vi "Filter Compare.vi"(10 "quantized filter":T1 {"mSRate_QSettings"."source" items=["Coef a/k"=0, "Coef b/v"=7, "Input"=1, "Output"=2, "Multiplicand"=3, "Product"=4, "Sum"=5, "Delay"=6, "Gain"=8]}, 11 "filter":T1 {"mSRate_QSettings"."source" items=["Coef a/k"=0, "Coef b/v"=7, "Input"=1, "Output"=2, "Multiplicand"=3, "Product"=4, "Sum"=5, "Delay"=6, "Gain"=8]}) -> (2 "phase (deg)":cluster{"Y":dbl[], "Y":dbl[]}[](graph), 3 "gain (dB)":cluster{"Y":dbl[], "Y":dbl[]}[](graph))   [LabVIEW 2011]
uses:
  <vilib>/addons/Digital Filter Design/_Objects.llb/DFD Filter Obj.ctl
  <vilib>/addons/Digital Filter Design/_Objects.llb/DFD Filter Coef.ctl
  <vilib>/addons/Digital Filter Design/_Objects.llb/DFD Filter Structure Type Selector.ctl
  <vilib>/addons/Digital Filter Design/_Objects.llb/dfd_Internal Quantization Settings.ctl
  <vilib>/addons/Digital Filter Design/_Objects.llb/dfd_Internal Quantization Srcs.ctl
  <vilib>/addons/Digital Filter Design/_Objects.llb/DFD Coef Norm Type.ctl
  <vilib>/addons/Digital Filter Design/_Objects.llb/DFD Phase Setting.ctl
  <vilib>/addons/Digital Filter Design/NI_DigFilterLicensed.lvlib
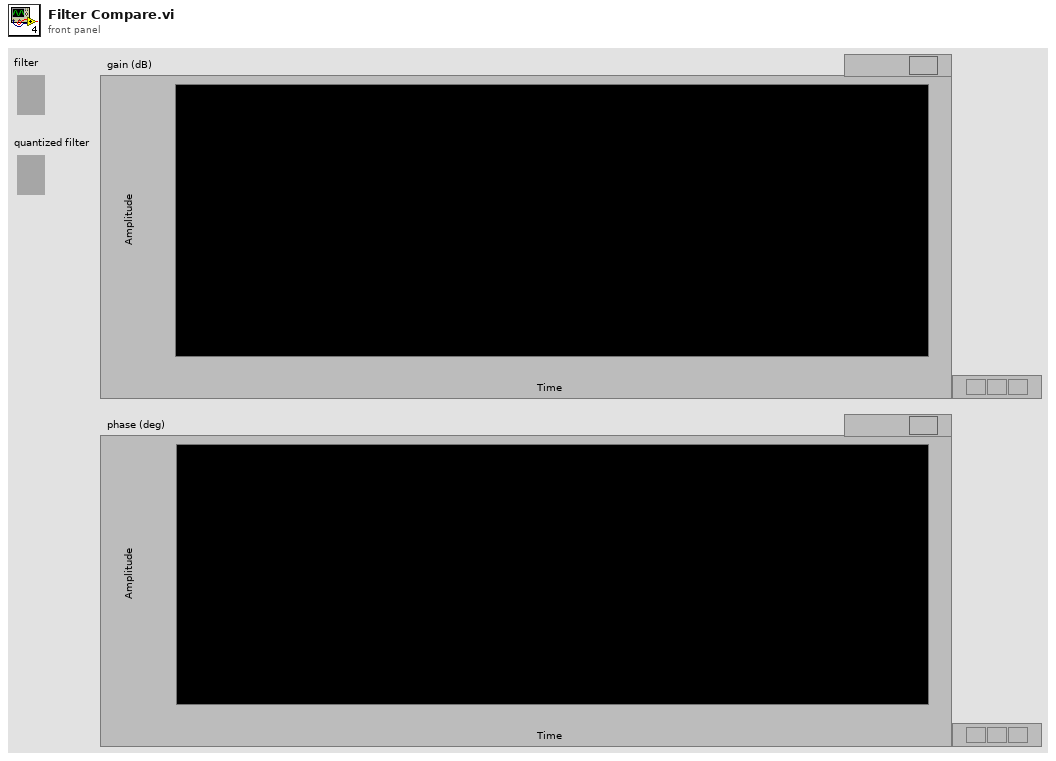
[diagram p1: front panel]
types:
  T1 = typedef "NI_DigFilterLicensed.lvlib/DFD Filter Obj.ctl" = cluster{"mSRate_Fs":dbl, "mSRate_Version":string, "mSRate_Comments":string, "mSRate_OrgCoef":T2, "mSRate_CurCoef":T2, "mSRate_Quantized?":bool, "mSRate_QCoef":T2, "mSRate_QSettings":T4[], "mSRate_Order":i32, "mSRate_Scaling":cluster{"mSRate_ScaleByPowerOf2?":bool, "mSRate_ScaleType":T6}}
  T2 = typedef "NI_DigFilterLicensed.lvlib/DFD Filter Coef.ctl" = cluster{"type":T3, "gain":dbl, "coef a (k)":dbl[], "coef b (v)":dbl[]}
  T3 = typedef "NI_DigFilterLicensed.lvlib/DFD Filter Structure Type Selector.ctl" = enum16{"Undefined", "FIR Direct Form", "FIR Direct Form Transposed", "FIR Symmetric", "FIR Antisymmetric", "IIR Direct Form I", "IIR Direct Form I Transposed", "IIR Direct Form II", "IIR Direct Form II Transposed", "IIR Cascaded Second Order Sections Form I", "IIR Cascaded Second Order Sections Form I Transposed", "IIR Cascaded Second Order Sections Form II", "IIR Cascaded Second Order Sections Form II Transposed", "Lattice Allpass (basic sections)", "Lattice Allpass (one multiplier sections)", "Lattice Allpass (normalized sections)", "Lattice AR (basic sections)", "Lattice AR (one multiplier sections)", "Lattice AR (normalized sections)", "Lattice MA (minimum phase)", "Lattice MA (maximum phase)", "Lattice ARMA (basic sections)", "Lattice ARMA (one multiplier sections)", "Lattice ARMA (normalized sections)"}
  T4 = typedef "NI_DigFilterLicensed.lvlib/dfd_Internal Quantization Settings.ctl" = cluster{"source":T5, "wl":i16, "iwl":i16, "overflow mode":enum16{"Saturation", "Wrap"}, "rounding mode":enum16{"Nearest", "Truncation"}, "signed?":bool}
  T5 = typedef "NI_DigFilterLicensed.lvlib/dfd_Internal Quantization Srcs.ctl" = u16
  T6 = typedef "NI_DigFilterLicensed.lvlib/DFD Coef Norm Type.ctl" = enum16{"No Norm", "Time Domain 1-Norm", "Time Domain 2-Norm", "Time Domain Inf-Norm"}
  T7 = typedef "NI_DigFilterLicensed.lvlib/DFD Phase Setting.ctl" = cluster{"unwrap? (F)":bool, "degree? (F)":bool}
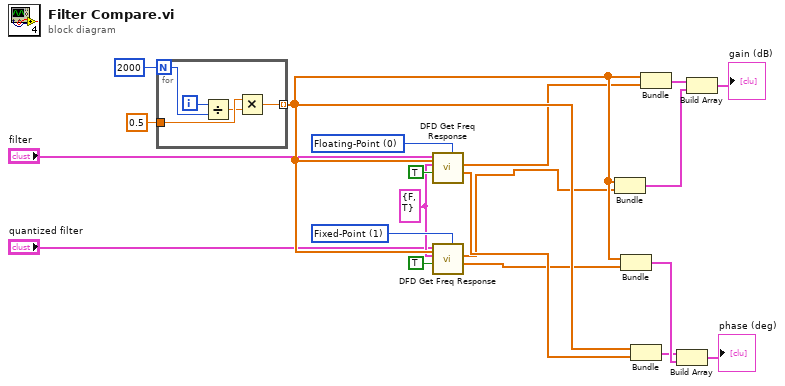
[diagram p0: block diagram]
diagram:
  w3 = T7 {"unwrap? (F)"=FALSE, "degree? (F)"=TRUE} ("phase view")
  w6 = u16 0 items=["Floating-Point", "Fixed-Point"] ("output option")
  w4 = u16 1 items=["Floating-Point", "Fixed-Point"] ("output option")
  n1 = for {
    N: 2000 -> [w24]
    tunnel: 0.5 -> [w23]
    tunnel: [w21] -> w16 mode=indexing
    i -> [w25]
    n2 = Divide(x=w25, y=w24) -> (x/y=w22:dbl)
    n3 = Multiply(x=w23, y=w22) -> (x*y=w21:dbl)
  }
  n4 = call <vilib>:"DFD Get Freq Response.vi"("output option"=w6, "freq points [Hz]"=w16, "dB on? (T)"=TRUE, "phase view"=w3, "filter in"="filter") -> ("phase"=w15:dbl[], "magnitude"=w10:dbl[])  [unwired: 3 in, 2 out]
  n5 = call <vilib>:"DFD Get Freq Response.vi"("output option"=w4, "freq points [Hz]"=w16, "dB on? (T)"=TRUE, "phase view"=w3, "filter in"="quantized filter") -> ("phase"=w8:dbl[], "magnitude"=w7:dbl[])  [unwired: 3 in, 2 out]
  n6 = Bundle(w16, "magnitude"=w7) -> (w17:cluster{dbl[], "magnitude":dbl[]})  [unwired: 1 in]
  n7 = Bundle(w16, "phase"=w8) -> (w18:cluster{dbl[], "phase":dbl[]})  [unwired: 1 in]
  n8 = Bundle(w16, "phase"=w15) -> (w14:cluster{dbl[], "phase":dbl[]})  [unwired: 1 in]
  n9 = Bundle(w16, "magnitude"=w10) -> (w11:cluster{dbl[], "magnitude":dbl[]})  [unwired: 1 in]
  n10 = Build Array(w14, w18) -> (→"phase (deg)":cluster{dbl[], "phase":dbl[]}[])
  n11 = Build Array(w11, w17) -> (→"gain (dB)":cluster{dbl[], "magnitude":dbl[]}[])
